vi "main.vi"() -> ()   [LabVIEW 2018]
uses:
  Control 12.ctl
  <vilib>/Instr/_visa.llb/VISA Configure Serial Port (Instr).vi
panel:
  in  "Tab Control":T1(tab)
  out "Temperatura (ºC)":dbl(slide) scale=0.0..50.0 scale format="%#.2f"
  out "Acceleròmetre":cluster{dbl, dbl, dbl}(graph)={-1477.92, 1162.76, -1186.5} caption="Waveform Chart - Dark"
  out "Giroscòpi":cluster{dbl, dbl, dbl}(graph)={-1477.92, 1162.76, -1186.5} caption="Waveform Chart - Dark"
  out "Magnetometre":cluster{dbl, dbl, dbl}(graph)={-4031.37, -986.16, -4204.69} caption="Waveform Chart - Dark"
  out "All Data":string
  in  "P_OFF 2":bool
  in  "START 2":bool
  in  "CONFIG SEL":bool
  in  "MOT SEL 3":bool
  out "Bobina 3":bool
  out "Bobina 2":bool
  out "Bobina 1":bool
  out "Motor":cluster{"Data Out":dbl, "Data Out":dbl}(graph) caption="Waveform Chart - Dark"
  in  "START 3":bool
  in  "P_OFF 3":bool
  in  "CONFIG SEL   2":bool
  in  "IMU SEL  3":bool
  out "Status":bool
  in  "Configuracions de VISA (UART)":T3={"stop bits (10: 1 bit)"=10, "baud rate "=115200, "parity (0:none)"=enum."None", "data bits (8)"=8, "Enable Termination\nChar"=TRUE, "Timeout "=1000, "VISA"="COM4", "termination char\n(0xA = '\\n' = LF) "=10} {"termination char\n(0xA = '\\n' = LF)" format="%.0x"; "data bits (8)" min=5 max=8 step=1; "stop bits (10: 1 bit)" items=["1.0"=10, "1.5"=15, "2.0"=20]}
  in  "P_OFF":bool
  in  "START":bool
  in  "MOT SEL":bool
  in  "IMU SEL":bool
  in  "Debug SEL 3":bool
  out "Error Source":string
  out "Motor DataString":string
  out "All Data":string
  in  "P_OFF 4":bool
  in  "START 4":bool
  out "VISA Buffer count":u32
  in  "MOCK CTRL":bool
  in  "Write a mock string":string=":0,0,0;0,0,0;0,0,0;0,0;"
  out "read buffer":string
  in  "Default":bool
  in  "CONFIG SEL   3":bool
  in  "MOT SEL 2":bool
  in  "IMU SEL  2":bool
  out "Error out Debug tab":errorcluster
  # "Angle"
  # "Fase"
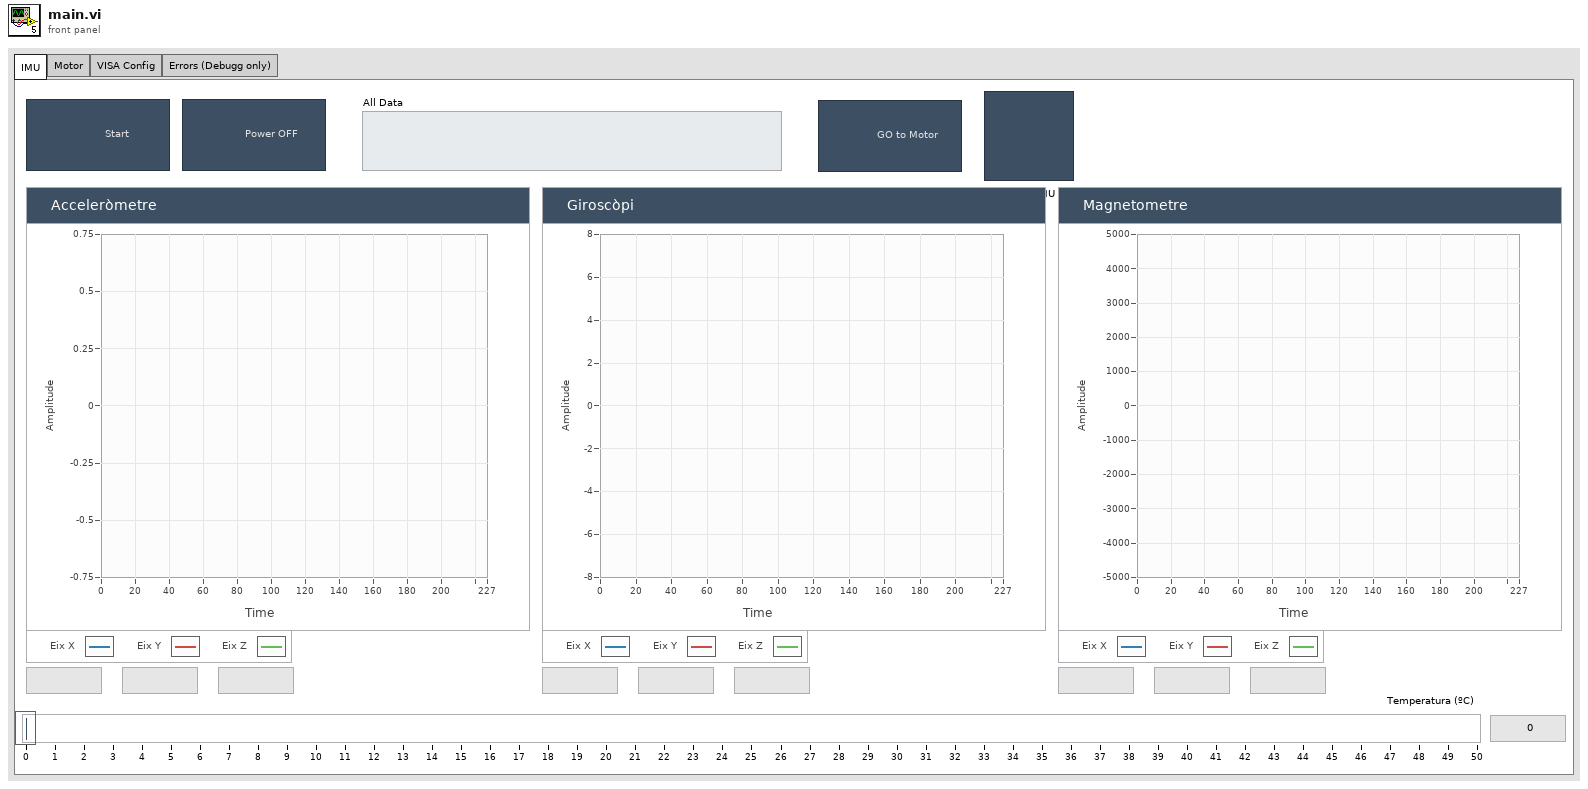
[diagram p1: front panel]
types:
  T1 = enum32{"IMU", "Motor", "VISA Config", "Errors (Debugg only)"}
  T2 = typedef "Control 12.ctl" = refnum<visa-resource-name>
  T3 = cluster{"stop bits (10: 1 bit)":u16, "baud rate ":u32, "parity (0:none)":enum16{"None", "Odd", "Even", "Mark", "Space"}, "data bits (8)":u16, "Enable Termination\nChar":bool, "Timeout ":u32, "VISA":T2, "termination char\n(0xA = '\\n' = LF) ":u8}
  T4 = cluster{"ShiftReg Right":cluster{"shift register right":string, "shift register right":string, "shift register right":string}, "ShiftReg Right":cluster{"shift register right":string, "shift register right":string, "shift register right":string}, "ShiftReg Right":cluster{"shift register right":string, "shift register right":string, "shift register right":string}, "ShiftReg RIGHT":cluster{"shift register right":string, "shift register right 2":string, "shift register right 3":string}, "read buffer":string}
  T5 = cluster{"P_OFF":bool, "P_OFF 2":bool, "P_OFF 3":bool, "P_OFF 4":bool}
  T6 = cluster{"START 4":bool, "START 2":bool, "START":bool, "START 3":bool}
  T7 = cluster{"POWER OFF OUT":bool, "STARTOUT":bool, "STARToutVAR":bool}
  T8 = cluster{"Angle (graus)":dbl, "Fase (#bobina)":dbl, "Temp":dbl}
  T9 = cluster{"Numeric":dbl, "Numeric":dbl, "Numeric":dbl}
  T10 = cluster{"ShiftReg Right":cluster{"shift register right":string, "shift register right":string, "shift register right":string}, "ShiftReg Right":cluster{"shift register right":string, "shift register right":string, "shift register right":string}, "ShiftReg Right":cluster{"shift register right":string, "shift register right":string, "shift register right":string}, "ShiftReg RIGHT":cluster{"shift register right":string, "shift register right 2":string, "shift register right 3":string}, "\n string out":string}
  T11 = cluster{"Angle (graus)":dbl, "Fase (#bobina)":dbl}
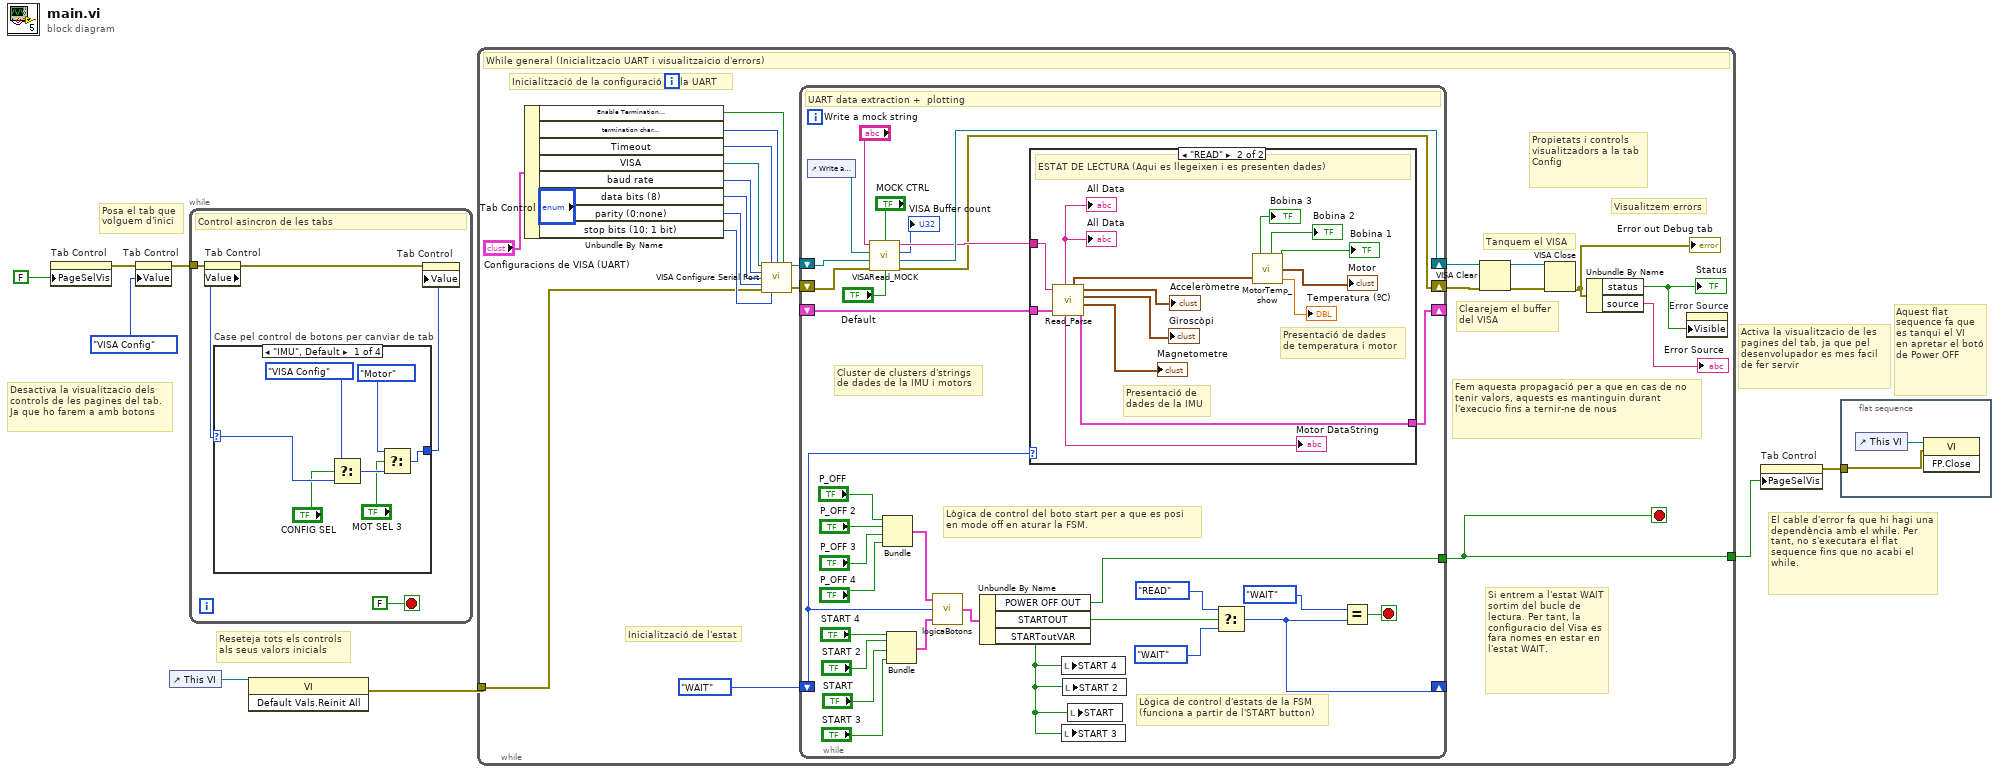
[diagram p0: block diagram]
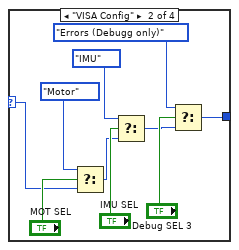
[diagram p2: hidden frame]
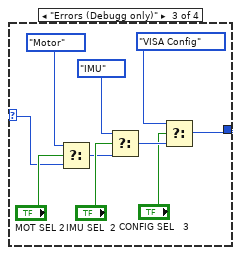
[diagram p3: hidden frame]
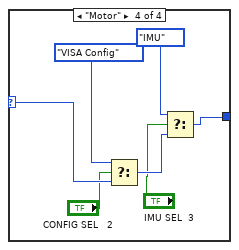
[diagram p4: hidden frame]
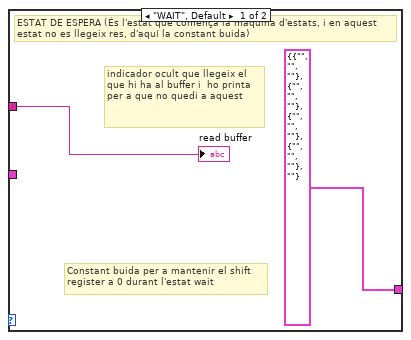
[diagram p5: hidden frame]
diagram:
  # "El cable d'error fa que hi hagi una dependència amb el while. Per tant, no s'executara el flat sequence fins que no acabi el while."
  # "Activa la visualitzacio de les pagines del tab, ja que pel desenvolupador es mes facil de fer servir"
  # "Aquest flat sequence fa que es tanqui el VI\nen apretar el botó de Power OFF"
  # "Desactiva la visualitzacio dels controls de les pagines del tab. Ja que ho farem a amb botons"
  # "Posa el tab que\nvolguem d'inici"
  # "Reseteja tots els controls \nals seus valors inicials"
  n1 = property on="Tab Control" class="TabCtl (strict)"("PageSelVis"=FALSE ("Page Selector Visible")) -> (error out=w3:errorcluster)  [unwired: 2 in, 1 out]
  n2 = property on="Tab Control" class="TabCtl (strict)"(error in=w3, "Value"=T1."VISA Config" ("t")) -> (error out=w2:errorcluster)  [unwired: 1 in, 1 out]
  n3 = control-ref of="This VI"() -> (w8:refnum<vi>)
  n4 = while {
    tunnel: w2 -> [w10]
    stop <- FALSE stop-if-true
    # "Control asincron de les tabs"
    n5 = property on="Tab Control" class="TabCtl (strict)"(error in=w10) -> (error out=w9:errorcluster, "Value"=w13:T1)  [unwired: 1 in, 1 out]
    n6 = case "Case pel control de botons per canviar de tab" shown="\"IMU\", Default" w13 {
      selector: w13 -> [w20 w23 w34 w46]
      tunnel: [w14 w21 w32 w41] -> w12
      frame "IMU", Default {
        n7 = Select(t=T1."VISA Config", s="CONFIG SEL", f=w20) -> (s? t:f=w17:T1)
        n8 = Select(t=T1."Motor", s="MOT SEL 3", f=w17) -> (s? t:f=w14:T1)
      }
      frame "VISA Config" {
        n9 = Select(t=T1."Motor", s="MOT SEL", f=w23) -> (s? t:f=w28:T1)
        n10 = Select(t=T1."IMU", s="IMU SEL", f=w28) -> (s? t:f=w22:T1)
        n11 = Select(t=T1."Errors (Debugg only)", s="Debug SEL 3", f=w22) -> (s? t:f=w21:T1)
      }
      frame "Errors (Debugg only)" {
        n12 = Select(t=T1."Motor", s="MOT SEL 2", f=w34) -> (s? t:f=w37:T1)
        n13 = Select(t=T1."IMU", s="IMU SEL  2", f=w37) -> (s? t:f=w33:T1)
        n14 = Select(t=T1."VISA Config", s="CONFIG SEL   3", f=w33) -> (s? t:f=w32:T1)
      }
      frame "Motor" {
        n15 = Select(t=T1."VISA Config", s="CONFIG SEL   2", f=w46) -> (s? t:f=w45:T1)
        n16 = Select(t=T1."IMU", s="IMU SEL  3", f=w45) -> (s? t:f=w41:T1)
      }
    }
    n17 = property on="Tab Control" class="TabCtl (strict)"(error in=w9, "Value"=w12) -> ()  [unwired: 1 in, 2 out]
  }
  n18 = invoke class="VI" method="Default Vals.Reinit All"(reference=w8) -> (error out=w4:errorcluster)  [unwired: 2 in, 2 out]
  n19 = while {
    tunnel: w4 -> [w49]
    tunnel: [w54] -> w5
    stop <- w54 stop-if-true
    # "Propietats i controls visualitzadors a la tab Config"
    # "Fem aquesta propagació per a que en cas de no tenir valors, aquests es mantinguin durant  l'execucio fins a ternir-ne de nous"
    # "Si entrem a l'estat WAIT sortim del bucle de lectura. Per tant, la configuracio del Visa es fara nomes en estar en l'estat WAIT."
    # "Inicialització de l'estat"
    # "Visualitzem errors"
    # "Clearejem el buffer\ndel VISA"
    # "Tanquem el VISA"
    # "Inicialització de la configuració de la UART"
    # "While general (Inicialitzacio UART i visualitzaicio d'errors)"
    n20 = Unbundle By Name("Configuracions de VISA (UART)") -> ("Enable Termination\nChar"=w62:bool, "termination char\n(0xA = '\\n' = LF)"=w55:u8, "Timeout"=w61:u32, "VISA"=w53:T2, "baud rate"=w52:u32, "data bits (8)"=w51:u16, "parity (0:none)"=w60:enum16{"None", "Odd", "Even", "Mark", "Space"}, "stop bits (10: 1 bit)"=w59:u16)
    n21 = call-poly "VISA Configure Serial Port"("VISA resource name"=w53, "timeout (10sec)"=w61, "termination char\n(0xA = '\\n' = LF)"=w55, "Enable Termination\nChar (T)"=w62, "baud rate (9600)"=w52, "data bits (8)"=w51, "parity (0:none)"=w60, "error in (no error)"=w49, "stop bits (10: 1 bit)"=w59) -> ("VISA resource name out"=w48:refnum<visa-resource-name>, "error out"=w68:errorcluster)  [unwired: 5 in]
    n22 = while {
      shift-right: [w95] -> _
      shift-left: enum16{"WAIT", "READ", ""}."WAIT" -> [w69]
      shift-right: [w72] -> w65
      shift-left: w68 -> [w79]
      shift-right: [w77] -> w67
      shift-left: w48 -> [w78]
      shift-right: [w98] -> _
      shift-left: _ -> [w97]
      tunnel: [w91] -> w54
      stop <- w96 stop-if-true
      # "Cluster de clusters d'strings\nde dades de la IMU i motors"
      # "Lògica de control d'estats de la FSM\n(funciona a partir de l'START button)"
      # "Lògica de control del boto start per a que es posi \nen mode off en aturar la FSM."
      # "UART data extraction +  plotting"
      n23 = control-ref of="Write a mock string"() -> (w75:refnum<vi>)
      n24 = call "VISARead_MOCK.vi"("MOCK CTRL"="MOCK CTRL", "mock string"="Write a mock string", "mock string reference"=w75, "Default"="Default", "VISA resource name in"=w78, "error in (no error)"=w79) -> ("string out"=w74:string, "return count"=→"VISA Buffer count":u32, "VISA Refnum out"=w77:refnum<visa-resource-name>, "error out"=w72:errorcluster)
      n25 = Bundle("P_OFF"="P_OFF", "P_OFF 2"="P_OFF 2", "P_OFF 3"="P_OFF 3", "P_OFF 4"="P_OFF 4") -> (w87:T5)  [unwired: 1 in]
      n26 = Bundle("START 4"="START 4", "START 2"="START 2", "START"="START", "START 3"="START 3") -> (w85:T6)  [unwired: 1 in]
      n27 = call "logicaBotons.vi"("Start IN's"=w85, "Entrada estat"=w69, "Power OFF IN's"=w87) -> ("Cluster"=w93:T7)
      n28 = Unbundle By Name(w93) -> ("POWER OFF OUT"=w91:bool, "STARTOUT"=w92:bool, "STARToutVAR"=w80:bool)
      n29 = case shown="\"READ\"" w69 {
        tunnel: w74 -> [w101 w111]
        tunnel: [T4 {"ShiftReg Right"={"shift register right"="", "shift register right"="", "shift register right"=""}, "ShiftReg Right"={"shift register right"="", "shift register right"="", "shift register right"=""}, "ShiftReg Right"={"shift register right"="", "shift register right"="", "shift register right"=""}, "ShiftReg RIGHT"={"shift register right"="", "shift register right 2"="", "shift register right 3"=""}, "read buffer"=""} w105] -> w98
        tunnel: w97 -> [_ w110]
        frame "WAIT", Default {
          # "Constant buida per a mantenir el shift\nregister a 0 durant l'estat wait"
          # "indicador ocult que llegeix el que hi ha al buffer i  ho printa per a que no quedi a aquest"
          # "ESTAT DE ESPERA (És l'estat que comença la maquina d'estats, i en aquest estat no es llegeix res, d'aquí la constant buida)"
          "read buffer" <- w101
        }
        frame "READ" {
          # "Presentació de \ndades de la IMU"
          # "Presentació de dades\nde temperatura i motor"
          # "ESTAT DE LECTURA (Aqui es llegeixen i es presenten dades)"
          n30 = call "Read_Parse.vi"("string in"=w111, "Cluster in"=w110) -> ("All Data"=→"All Data" →"All Data":string, "Motor DataString"=→"Motor DataString":string, "DADES"=w107:T8, "Acceleròmetre"=→"Acceleròmetre":T9, "Giroscopi"=→"Giroscòpi":T9, "Magnetometre"=→"Magnetometre":T9, "Cluster out"=w105:T10)  [unwired: 2 in]
          n31 = call "MotorTemp_show.vi"("DADES"=w107) -> ("Temp"=→"Temperatura (ºC)":dbl, "Cluster"=→"Motor":T11, "Button 3"=→"Bobina 1":bool, "Button 2"=→"Bobina 2":bool, "Button"=→"Bobina 3":bool)  [unwired: 1 in]
        }
      }
      n32 = local write "START 4"(w80) -> ()
      n33 = local write "START 3"(w80) -> ()
      n34 = local write "START 2"(w80) -> ()
      n35 = local write "START"(w80) -> ()
      n36 = Select(t=enum16{"WAIT", "READ", ""}."READ", s=w92, f=enum16{"WAIT", "READ", ""}."WAIT") -> (s? t:f=w95:enum16{"WAIT", "READ", ""})
      n37 = Equal?(x=enum16{"WAIT", "READ", ""}."WAIT", y=w95) -> (x = y?=w96:bool)
    }
    n38 = VISA Clear(VISA resource name=w67, error in (no error)=w65) -> (VISA resource name out=w66:refnum<visa-resource-name>, error out=w64:errorcluster)
    n39 = VISA Close(VISA resource name=w66, error in (no error)=w64) -> (error out=w56:errorcluster)
    "Error out Debug tab" <- w56
    n40 = Unbundle By Name(w56) -> ("status"=w57:bool, "source"=→"Error Source":string)
    "Status" <- w57
    n41 = property on="Error Source" class="Str"("Visible"=w57) -> ()  [unwired: 2 in, 2 out]
  }
  n42 = property on="Tab Control" class="TabCtl (strict)"("PageSelVis"=w5) -> (error out=w1:errorcluster)  [unwired: 2 in, 1 out]
  n43 = flat-sequence {
    tunnel: w1 -> [w117]
    frame #0 {
      n44 = control-ref of="This VI"() -> (w118:refnum<vi>)
      n45 = invoke class="VI" method="FP.Close"(reference=w118, error in=w117) -> ()  [unwired: 1 in, 3 out]
    }
  }
